vi "打开通信连接.vi"(8 "error in (no error)":errorcluster, 11 "串口通信类 in":refnum<class "串口通信类.lvclass">) -> (0 "error out":errorcluster, 3 "串口通信类 out":refnum<class "串口通信类.lvclass">)   [LabVIEW 2015, in "串口通信类.lvclass"]
uses:
  <vilib>/Instr/_visa.llb/VISA Configure Serial Port (Instr).vi
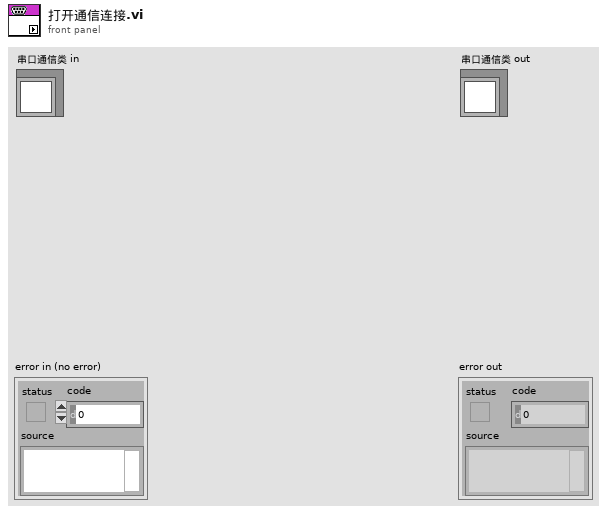
[diagram p1: front panel]
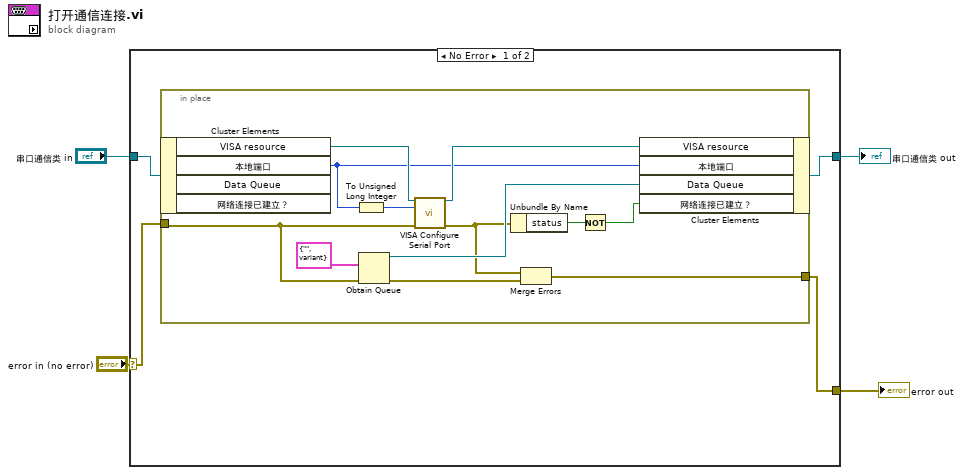
[diagram p0: block diagram]
diagram:
  n1 = case shown="No Error" "error in (no error)" {
    selector: "error in (no error)" -> [w8 w22]
    tunnel: [w7 w22] -> w3
    tunnel: "串口通信类 in" -> [w6 w21]
    tunnel: [w5 w21] -> w1
    frame No Error {
      n2 = in-place "In Place Element Structure" {
        in-place-border: w8 -> [w15]
        in-place-border: [w13] -> w7
        n3 = in-place-cluster #1(w6) -> ("VISA resource"=w19:refnum<visa-resource-name>, "本地端口"=w17:u16)  [unwired: 2 out]
        n4 = To Unsigned Long Integer(number=w17) -> (unsigned 32bit integer=w20:u32)
        n5 = Obtain Queue(element data type=cluster{string, variant} {"", variant} ("cluster"), error in (no error)=w15) -> (queue out=w12:refnum<queue>, error out=w14:errorcluster)  [unwired: 3 in, 1 out]
        n6 = call-poly "VISA Configure Serial Port"("VISA resource name"=w19, "baud rate (9600)"=w20, "error in (no error)"=w15) -> ("VISA resource name out"=w18:refnum<visa-resource-name>, "error out"=w11:errorcluster)  [unwired: 11 in]
        n7 = Unbundle By Name(w11) -> ("status"=w10:bool)
        n8 = Merge Errors(w11, w14) -> (w13:errorcluster)
        n9 = Not(x=w10) -> (.not. x?=w9:bool)
        n10 = in-place-cluster #1("VISA resource"=w18, "本地端口"=w17, "Data Queue"=w12, "网络连接已建立？"=w9) -> (w5:refnum<class "串口通信类.lvclass">)
      }
    }
    frame Error {
    }
  }
  "error out" <- w3
  "串口通信类 out" <- w1
